vi "PathFilterTest.vi"(11 "error in":errorcluster) -> (15 "error out":errorcluster)   [LabVIEW 2023, in "TestVIs.lvlib"]
uses:
  TestVIs.lvlib
  <vilib>/addons/_JKI Toolkits/Caraya/classes/Assert/Assert Equal Value_Variant.vi
  <vilib>/addons/_JKI Toolkits/Caraya/classes/Test/Test.lvclass
  Library/Unit Testing CA1.lvlib
  <vilib>/addons/_JKI Toolkits/Caraya/classes/Assert/Assert.lvclass
panel:
  # "PATH FILTER TEST"
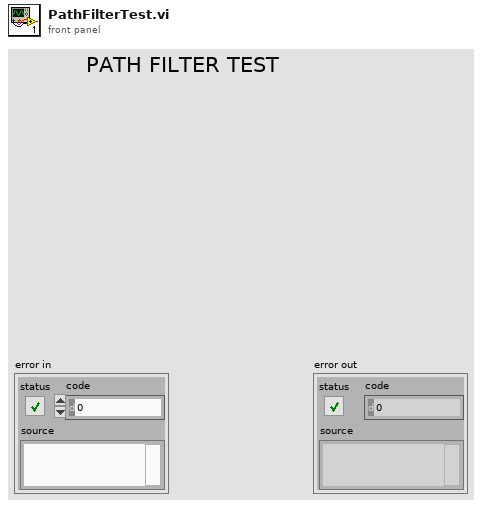
[diagram p1: front panel]
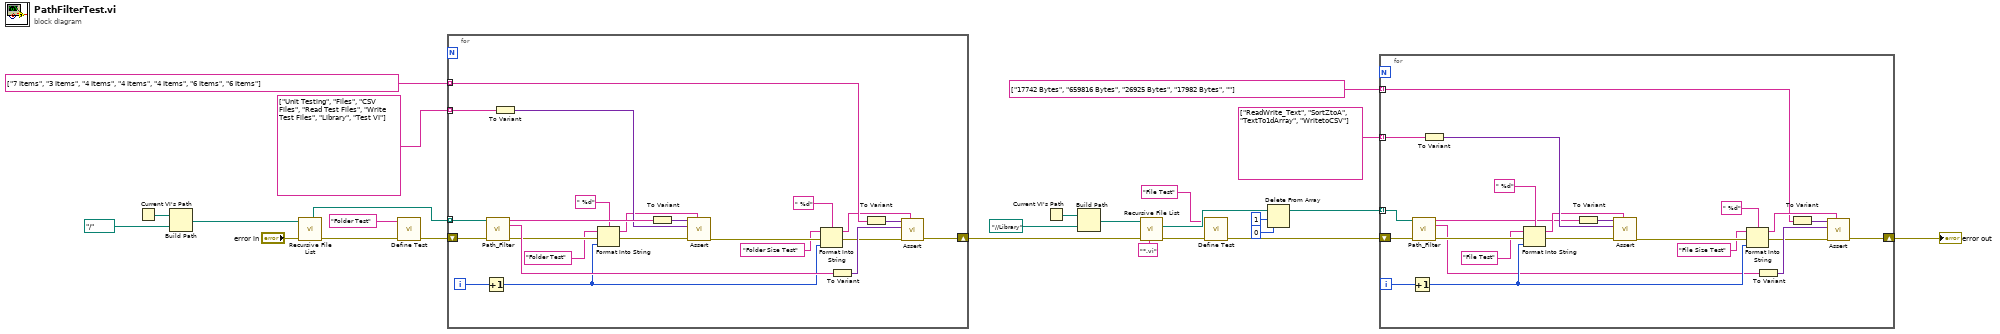
[diagram p0: block diagram]
diagram:
  n1 = Current VI's Path() -> (path=w12:path)
  n2 = Build Path(base path=w12, name or relative path=path "../..") -> (appended path=w9:path)
  n3 = call <vilib>:"Recursive File List.vi"("error in (no error)"="error in", "Folder Path"=w9) -> ("error out"=w10:errorcluster, "All Folders"=w8:path[])  [unwired: 5 in, 3 out]
  n4 = call <vilib>:"Define Test.vi"("error in (no error)"=w10, "Label (VI Title)"="Folder Test") -> ("error out"=w21:errorcluster)  [unwired: 8 in, 1 out]
  n5 = for {
    tunnel: w8 -> [w48] mode=indexing
    shift-right: [w41] -> w14
    shift-left: w21 -> [w47]
    tunnel: string[] ["Unit Testing", "Files", "CSV Files", "Read Test Files", "Write Test Files", "Library", "Test VI"] ("Array") -> [w45] mode=indexing
    tunnel: string[] ["7 Items", "3 Items", "4 Items", "4 Items", "4 Items", "6 Items", "6 Items"] ("Array 2") -> [w38] mode=indexing
    i -> [w34]
    n6 = Increment(x=w34) -> (x+1=w28:i32)
    n7 = call "Path_Filter.vi"("path"=w48, "error in"=w47) -> ("File/Folder Name"=w46:string, "Size"=w40:string, "error out"=w37:errorcluster)  [unwired: 11 in]
    n8 = To Variant(anything=w45) -> (Variant=w44:variant)
    n9 = Format Into String(format string=" %d", initial string="Folder Test" ("Label"), error in=w37, w28) -> (resulting string=w32:string, error out=w36:errorcluster)
    n10 = To Variant(anything=w46) -> (Variant=w43:variant)
    n11 = call-poly <vilib>:"Assert.vi"("Label"=w32, "error in (no error)"=w36, "Y"=w44, "X"=w43) -> ("error out"=w30:errorcluster)  [unwired: 6 in, 1 out]
    n12 = Format Into String(format string=" %d", initial string="Folder Size Test" ("Label"), error in=w30, w28) -> (resulting string=w27:string, error out=w26:errorcluster)
    n13 = To Variant(anything=w40) -> (Variant=w39:variant)
    n14 = To Variant(anything=w38) -> (Variant=w42:variant)
    n15 = call-poly <vilib>:"Assert.vi"("Label"=w27, "error in (no error)"=w26, "Y"=w39, "X"=w42) -> ("error out"=w41:errorcluster)  [unwired: 6 in, 1 out]
  }
  n16 = Current VI's Path() -> (path=w7:path)
  n17 = Build Path(base path=w7, name or relative path=path "../../Library") -> (appended path=w5:path)
  n18 = call <vilib>:"Recursive File List.vi"("pattern"="*.vi", "error in (no error)"=w14, "Folder Path"=w5) -> ("error out"=w17:errorcluster, "All Files in Dir"=w20:path[])  [unwired: 4 in, 3 out]
  n19 = call <vilib>:"Define Test.vi"("error in (no error)"=w17, "Label (VI Title)"="File Test") -> ("error out"=w16:errorcluster)  [unwired: 8 in, 1 out]
  n20 = Delete From Array(array=w20, length=1, index=0) -> (array with subset deleted=w3:path[])  [unwired: 1 out]
  n21 = for {
    tunnel: w3 -> [w71] mode=indexing
    shift-right: [w66] -> w13
    shift-left: w16 -> [w70]
    tunnel: string[] ["17742 Bytes", "659816 Bytes", "26925 Bytes", "17982 Bytes", ""] ("Array 2") -> [w49] mode=indexing
    tunnel: string[] ["ReadWrite_Text", "SortZtoA", "TextTo1dArray", "WritetoCSV"] ("Array") -> [w50] mode=indexing
    i -> [w61]
    n22 = Increment(x=w61) -> (x+1=w55:i32)
    n23 = call "Path_Filter.vi"("path"=w71, "error in"=w70) -> ("File/Folder Name"=w51:string, "Size"=w53:string, "error out"=w64:errorcluster)  [unwired: 11 in]
    n24 = To Variant(anything=w50) -> (Variant=w69:variant)
    n25 = Format Into String(format string=" %d", initial string="File Test" ("Label"), error in=w64, w55) -> (resulting string=w59:string, error out=w63:errorcluster)
    n26 = To Variant(anything=w51) -> (Variant=w68:variant)
    n27 = call-poly <vilib>:"Assert.vi"("Label"=w59, "error in (no error)"=w63, "Y"=w69, "X"=w68) -> ("error out"=w57:errorcluster)  [unwired: 6 in, 1 out]
    n28 = Format Into String(format string=" %d", initial string="File Size Test" ("Label"), error in=w57, w55) -> (resulting string=w52:string, error out=w54:errorcluster)
    n29 = To Variant(anything=w53) -> (Variant=w65:variant)
    n30 = To Variant(anything=w49) -> (Variant=w67:variant)
    n31 = call-poly <vilib>:"Assert.vi"("Label"=w52, "error in (no error)"=w54, "Y"=w65, "X"=w67) -> ("error out"=w66:errorcluster)  [unwired: 6 in, 1 out]
  }
  "error out" <- w13
